vi "Protocol.Claim Addresses.vi"(8 "error in":errorcluster, 10 "J1939 Main Configuration":T1, 11 "Parameters in":T8={"XNET Settings"={"Database"="", "Cluster"="", "Port"="", "Baud rate [Bd]"=0, "Termination"=0, "Incoming Rate"=0, "Outcoming Rate"=1, "Write Decimation"=1}, "Data"=[], "DTCs"=[], "Sim Addresses LUT"=variant, "Data Table LUT"=variant, "MonitorTool.Network"={"Address"=0, "Name"=0}, "Name"=""} {"MonitorTool.Network"."Name" format="%.0x"; "DTCs"."Data"."DM1 Ref"."Data Reference" format="%.0x"; "DTCs"."Data"."DM1 Enable Ref"."Data Reference" format="%.0x"; "DTCs"."Data"."DM2 Ref"."Data Reference" format="%.0x"; "DTCs"."Data"."DM2 Enable Ref"."Data Reference" format="%.0x"; "Data"."Timing.Refs"."Data Reference" format="%.0x"; "Data"."Network"."Name" format="%.0x"; "Data"."IncomingRefs"."Data Reference" format="%.0x"; "Data"."OutgoingRefs"."Data Reference" format="%.0x"; "XNET Settings"."Termination" items=["Off", "On"]}) -> (0 "error out":errorcluster, 3 "output cluster":T1)   [LabVIEW 2015, in "J1939 Addon Engine.lvlib"]
uses:
  J1939 Addon Engine.lvlib
  Types/Protocol.Configuration.ctl
  <vilib>/NI/NIVS Addon Network Comm/Engine/VeriStand Comm.lvclass
  <vilib>/NI/NIVS Inline Async API/_VS Inline Async API/Process/Process.lvclass
  Types/Protocol.Refs.ctl
  Shared/J1939 Utilities/Types/CAN Outgoing Message Cluster.ctl
  Types/Protocol.RQST Lookup Table Reference.ctl
  Types/Protocol.Address Table Reference.ctl
  Types/Protocol.XNET Settings.ctl
  <vilib>/NI/NIVS Inline Async API/_Data Access Engine/Data Access Engine/Types/Read.DVR.ctl
  <vilib>/NI/NIVS Inline Async API/_Data Access Engine/Access Type Classes/Read/Read.lvclass
  <vilib>/NI/NIVS Inline Async API/_Data Access Engine/Data Access Engine/Types/Write.DVR.ctl
  <vilib>/NI/NIVS Inline Async API/_Data Access Engine/Access Type Classes/Write/Write.lvclass
  Types/Protocol.App Settings.ctl
  Shared/Types/XNET Settings.ctl
  Types/Protocol.XNET Refs.ctl
  <vilib>/NI Veristand/Custom Device API/Block Data Reference.ctl
  <vilib>/NI Veristand/Custom Device API/Data Reference.ctl
  Shared/Types/Monitor Settings.ctl
  Types/Engine.DTC Settings.ctl
  Shared/Types/Compiled Simulated Settings.ctl
  Types/Engine.DTC FIFOs.ctl
  <resource>/objmgr/xnet.rc
  <vilib>/NI Veristand/Custom Device Tools/Custom Device Utility Library/Custom Device Utility Library.lvlib
  Shared/J1939 Utilities/J1939 Utilities.lvlib
  Shared/J1939 Addon Shared.lvlib
  <vilib>/NI VeriStand/Custom Device API/Custom Device API.lvlib
  <vilib>/NI/NIVS Inline Async API/_Data Access Engine/Data Access Engine/Data Access Engine.lvclass
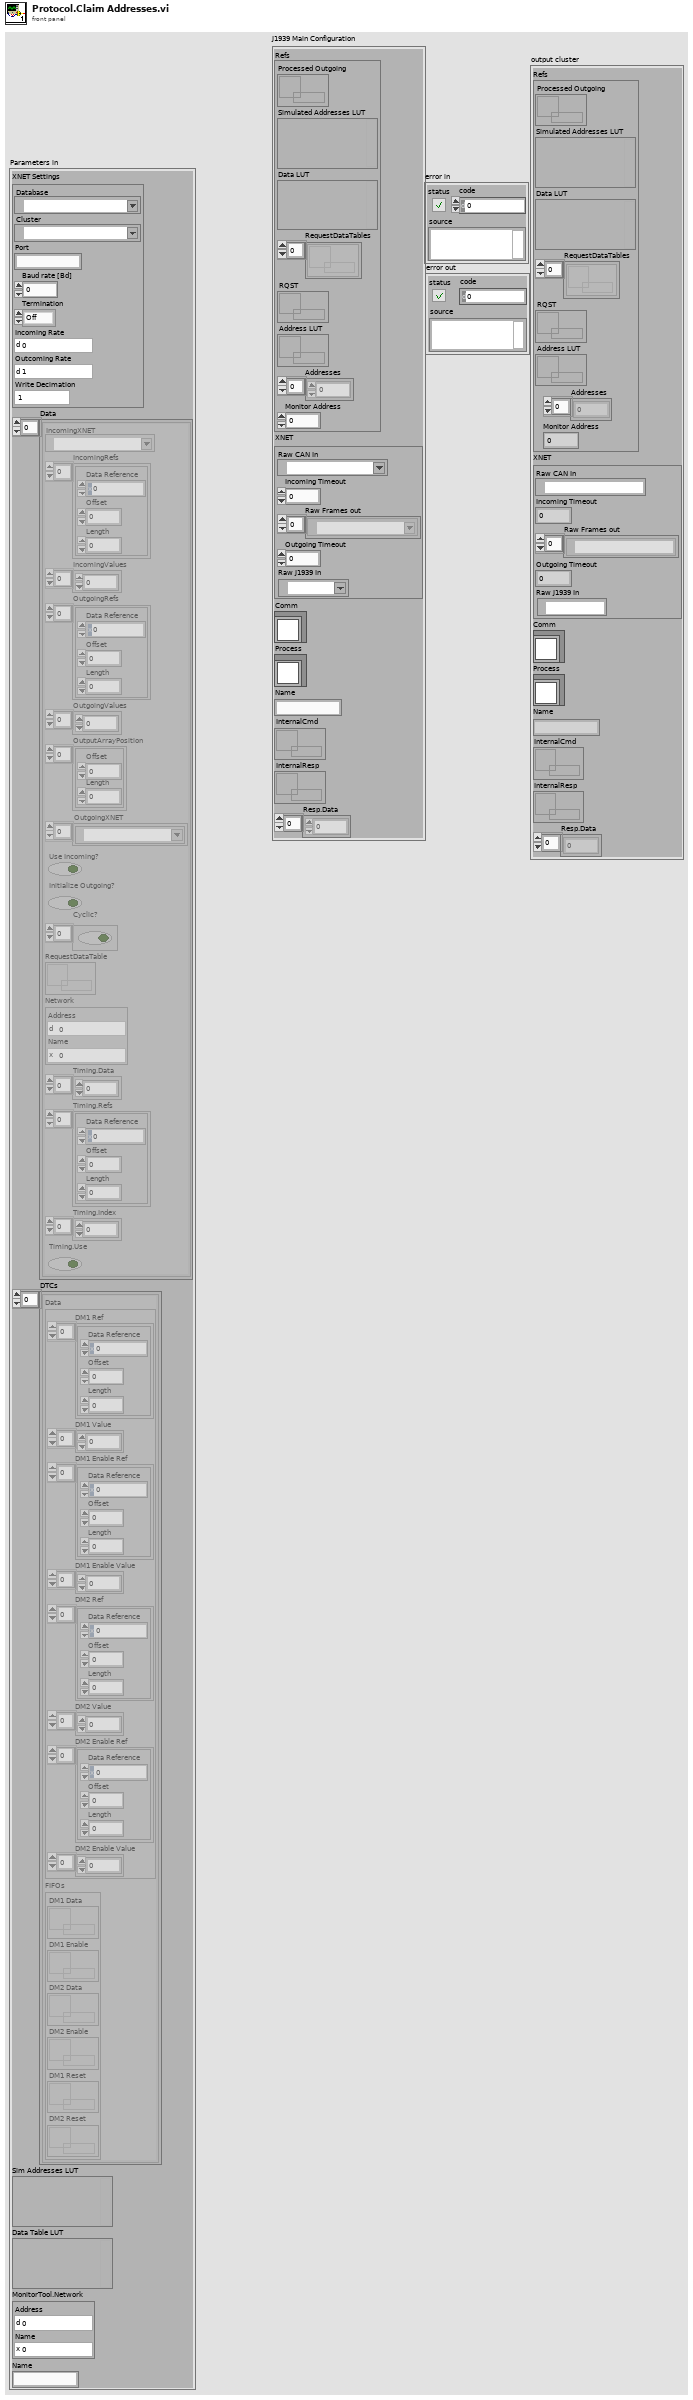
[diagram p1: front panel]
types:
  T1 = typedef "J1939 Addon Engine.lvlib/Protocol.Configuration.ctl" = cluster{"Refs":T2, "XNET":T5, "Comm":refnum<class "VeriStand Comm.lvclass">, "Process":refnum<class "Process.lvclass">, "Name":string, "InternalCmd":T6, "InternalResp":T7, "Resp.Data":dbl[]}
  T2 = typedef "J1939 Addon Engine.lvlib/Protocol.Refs.ctl" = cluster{"Processed Outgoing":refnum<queue>, "Simulated Addresses LUT":variant, "Data LUT":variant, "RequestDataTables":refnum<k33>[], "RQST":T3, "Address LUT":T4, "Addresses":u8[], "Monitor Address":u8}
  T3 = typedef "J1939 Addon Engine.lvlib/Protocol.RQST Lookup Table Reference.ctl" = refnum<data-value>
  T4 = typedef "J1939 Addon Engine.lvlib/Protocol.Address Table Reference.ctl" = refnum<data-value>
  T5 = typedef "J1939 Addon Engine.lvlib/Protocol.XNET Settings.ctl" = cluster{"Raw CAN In":refnum<k21>, "Incoming Timeout":u32, "Raw Frames out":refnum<k21>[], "Outgoing Timeout":u32, "Raw J1939 In":refnum<k21>}
  T6 = typedef "Data Access Engine.lvlib/Data Access Engine.lvclass/Read.DVR.ctl" = refnum<data-value>
  T7 = typedef "Data Access Engine.lvlib/Data Access Engine.lvclass/Write.DVR.ctl" = refnum<data-value>
  T8 = typedef "J1939 Addon Engine.lvlib/Protocol.App Settings.ctl" = cluster{"XNET Settings":T9, "Data":T10[], "DTCs":T14[], "Sim Addresses LUT":variant, "Data Table LUT":variant, "MonitorTool.Network":T13, "Name":string}
  T9 = typedef "J1939 Addon Shared.lvlib/XNET Settings.ctl" = cluster{"Database":refnum<k21>, "Cluster":refnum<k21>, "Port":string, "Baud rate [Bd]":u32, "Termination":u32, "Incoming Rate":u32, "Outcoming Rate":u32, "Write Decimation":u32}
  T10 = typedef "J1939 Addon Engine.lvlib/Protocol.XNET Refs.ctl" = cluster{"IncomingXNET":refnum<k21>, "IncomingRefs":T11[], "IncomingValues":dbl[], "OutgoingRefs":T11[], "OutgoingValues":dbl[], "OutputArrayPosition":cluster{"Offset":u32, "Length":u32}[], "OutgoingXNET":refnum<k21>[], "Use Incoming?":bool, "Initialize Outgoing?":bool, "Cyclic?":bool[], "RequestDataTable":refnum<k33>, "Network":T13, "Timing.Data":dbl[], "Timing.Refs":T11[], "Timing.Index":i32[], "Timing.Use":bool}
  T11 = typedef "Custom Device API.lvlib/Block Data Reference.ctl" = cluster{"Data Reference":T12, "Offset":u64, "Length":u64}
  T12 = typedef "Custom Device API.lvlib/Data Reference.ctl" = i32
  T13 = typedef "J1939 Addon Shared.lvlib/Monitor Settings.ctl" = cluster{"Address":u8, "Name":u64}
  T14 = typedef "J1939 Addon Engine.lvlib/Engine.DTC Settings.ctl" = cluster{"Data":T15, "FIFOs":T16}
  T15 = typedef "J1939 Addon Shared.lvlib/Compiled Simulated Settings.ctl" = cluster{"DM1 Ref":T11[], "DM1 Value":dbl[], "DM1 Enable Ref":T11[], "DM1 Enable Value":dbl[], "DM2 Ref":T11[], "DM2 Value":dbl[], "DM2 Enable Ref":T11[], "DM2 Enable Value":dbl[]}
  T16 = typedef "J1939 Addon Engine.lvlib/Engine.DTC FIFOs.ctl" = cluster{"DM1 Data":refnum<k33>, "DM1 Enable":refnum<k33>, "DM2 Data":refnum<k33>, "DM2 Enable":refnum<k33>, "DM1 Reset":refnum<k33>, "DM2 Reset":refnum<k33>}
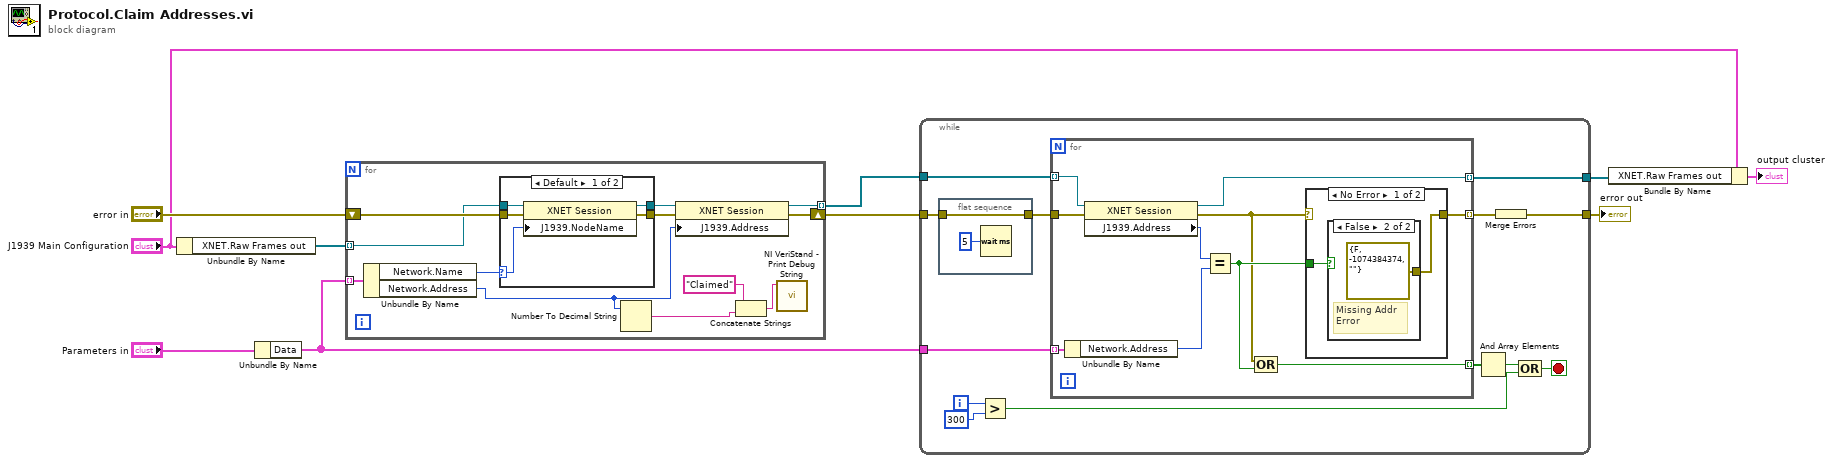
[diagram p0: block diagram]
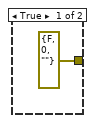
[diagram p2: hidden frame]
diagram:
  n1 = Unbundle By Name("J1939 Main Configuration") -> ("XNET.Raw Frames out"=w8:refnum<k21>[])
  n2 = Unbundle By Name("Parameters in") -> ("Data"=w6:T10[])
  n3 = for {
    shift-right: [w21] -> w10
    shift-left: "error in" -> [w22]
    tunnel: w6 -> [w18] mode=indexing
    tunnel: w8 -> [w16] mode=indexing
    tunnel: [w15] -> w9 mode=indexing
    n4 = Unbundle By Name(w18) -> ("Network.Name"=w17:u64, "Network.Address"=w14:u8)
    n5 = case shown="Default" w17 {
      selector: w17 -> [w25 _]
      tunnel: w16 -> [w27 w28]
      tunnel: w22 -> [w26 w29]
      tunnel: [w24 w29] -> w20
      tunnel: [w23 w28] -> w19
      frame Default {
        n6 = property class="XNET Session"(reference=w27, error in=w26, "J1939.NodeName"=w25) -> (reference out=w23:refnum<k21>, error out=w24:errorcluster)
      }
      frame 0 {
      }
    }
    n7 = Number To Decimal String(number=w14) -> (decimal integer string=w13:string)  [unwired: 1 in]
    n8 = property class="XNET Session"(reference=w19, error in=w20, "J1939.Address"=w14) -> (reference out=w15:refnum<k21>, error out=w21:errorcluster)
    n9 = Concatenate Strings("Claimed" ("Message"), w13) -> (w11:string)
    n10 = call <vilib>:"NI VeriStand - Print Debug String.vi"("Message"=w11) -> ()  [unwired: 10 in, 1 out]
  }
  n11 = while {
    tunnel: w10 -> [w39]
    tunnel: [w41] -> w4
    tunnel: w9 -> [w31]
    tunnel: w6 -> [w32]
    tunnel: [w30] -> w2
    i -> [w37]
    stop <- w33 stop-if-true
    n12 = flat-sequence {
      tunnel: [w44] -> w40
      tunnel: w39 -> [w44]
      frame #0 {
        n13 = Wait (ms)(milliseconds to wait=u32 5) -> ()  [unwired: 1 out]
      }
    }
    n14 = Greater?(x=w37, y=300) -> (0:w34:bool)
    n15 = for {
      tunnel: w40 -> [w54]
      tunnel: [w53] -> w42 mode=indexing
      tunnel: w31 -> [w52] mode=indexing
      tunnel: [w51] -> w36 mode=indexing
      tunnel: w32 -> [w50] mode=indexing
      tunnel: [w45] -> w30 mode=indexing
      n16 = Unbundle By Name(w50) -> ("Network.Address"=w49:u8)
      n17 = property class="XNET Session"(reference=w52, error in=w54) -> (reference out=w45:refnum<k21>, error out=w47:errorcluster, "J1939.Address"=w46:u8)
      n18 = Equal?(x=w46, y=w49) -> (x = y?=w48:bool)
      n19 = Compound Arithmetic op=OR(w47, w48) -> (w51:bool)
      n20 = case shown="No Error" w47 {
        selector: w47 -> [_ w59]
        tunnel: w48 -> [w56 _]
        tunnel: [w55 w59] -> w53
        frame No Error {
          n21 = case shown="False" w56 {
            tunnel: [errorcluster {"status"=FALSE, "code"=0, "source"=""} ("error out") errorcluster {"status"=FALSE, "code"=-1074384374, "source"=""} ("error out")] -> w55
            frame True {
            }
            frame False {
              # "Missing Addr\nError"
            }
          }
        }
        frame Error {
        }
      }
    }
    n22 = And Array Elements(Boolean array=w36) -> (logical AND=w35:bool)
    n23 = Merge Errors(w42) -> (w41:errorcluster)
    n24 = Compound Arithmetic op=OR(w35, w34) -> (w33:bool)
  }
  "error out" <- w4
  n25 = Bundle By Name(cluster="J1939 Main Configuration", "XNET.Raw Frames out"=w2) -> (→"output cluster":T1)
